vi "Write B.vi"(8 "error in (no error)":errorcluster, 10 "B":dbl, 11 "Linear in":refnum<class "Linear.lvclass">) -> (0 "error out":errorcluster, 3 "Linear out":refnum<class "Linear.lvclass">)   [LabVIEW 2020, in "Data Generators.lvlib" / "Linear.lvclass"]
uses:
  Linear.lvclass
  Linear.lvclass/Linear.ctl
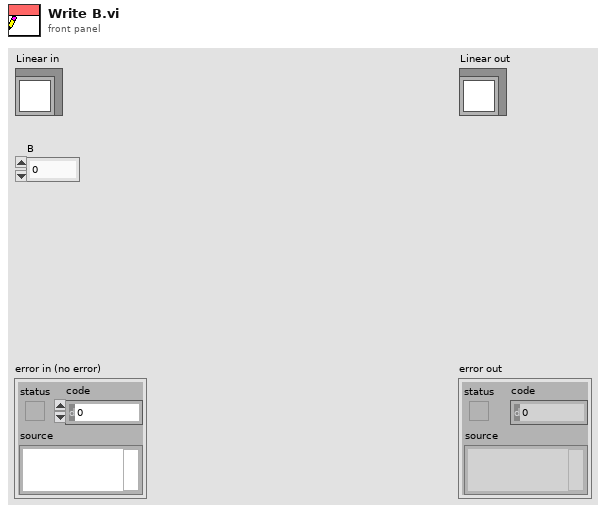
[diagram p1: front panel]
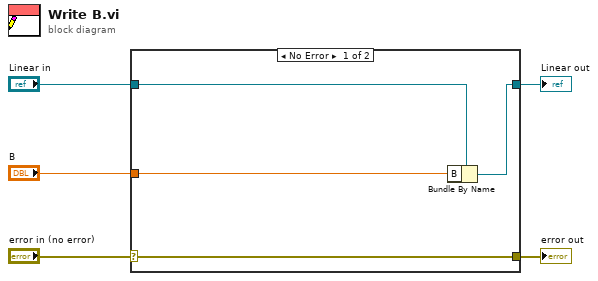
[diagram p0: block diagram]
diagram:
  n1 = case shown="No Error" "error in (no error)" {
    selector: "error in (no error)" -> [w9 w10]
    tunnel: [w9 w10] -> w4
    tunnel: [w7 w11] -> w2
    tunnel: "Linear in" -> [w8 w11]
    tunnel: "B" -> [w6 _]
    frame No Error {
      n2 = Bundle By Name(cluster=w8, "B"=w6) -> (w7:refnum<class "Linear.lvclass">)
    }
    frame Error {
    }
  }
  "error out" <- w4
  "Linear out" <- w2
